vi "niRFUtil MT LTE Composite Equalization.vi"(6 "Threshold":sgl, 8 "error in (no error)":errorcluster, 9 "OFDM symbol to skip":i32, 10 "Ideal signal":csg[][](array[numeric]), 11 "Received signal":csg[][](array[numeric])) -> (0 "error out":errorcluster, 2 "Equalizer coefficients":csg[](array[numeric]), 3 "Equalized signal":csg[][](array[numeric]))   [LabVIEW 2015, in "niRFUtil.lvlib"]
uses:
  niRFUtil.lvlib
  Utilities/niRFAMT.dll
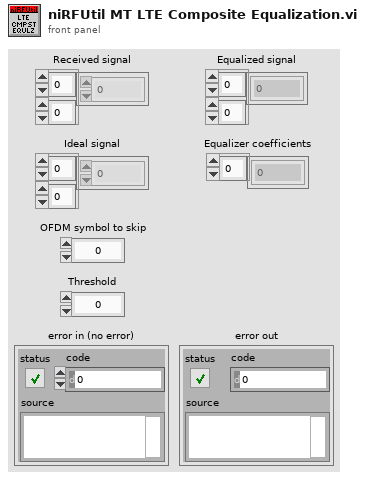
[diagram p1: front panel]
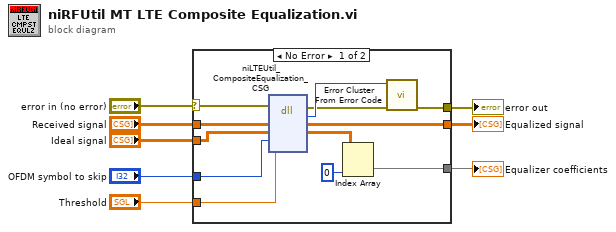
[diagram p0: block diagram]
diagram:
  n1 = case shown="No Error" "error in (no error)" {
    selector: "error in (no error)" -> [w9 w21]
    tunnel: "Received signal" -> [w20 _]
    tunnel: "Ideal signal" -> [w19 _]
    tunnel: "OFDM symbol to skip" -> [w18 _]
    tunnel: "Threshold" -> [w17 _]
    tunnel: [w16 _] -> w4
    tunnel: [w13 _] -> w3
    tunnel: [w10 w21] -> w2
    frame No Error {
      n2 = dll-call lib="C:/Perforce/semoore-sales/Customers/NATI-3813/Noise Floor/LV Filters/ParallelComplexFilterRFUtil/niRFUtil/MT/Utilities/niRFAMT.*" fn="niLTEUtil_CompositeEqualization_CSG"(error in=w9, "Received signal"=w20, "Ideal signal"=w19, "OFDM symbol to skip"=w18, "Threshold"=w17) -> (error out=w11:errorcluster, "return type"=w12:i32, "Received signal"=w16:csg[][], "Ideal signal"=w14:csg[][])  [unwired: 4 in, 1 out]
      n3 = Index Array(array=w14, index (col)=0 ("disabled index (col)")) -> (element=w13:csg[])  [unwired: 1 in]
      n4 = call <vilib>:"Error Cluster From Error Code.vi"("error in (no error)"=w11, "error code (0)"=w12) -> ("error out"=w10:errorcluster)  [unwired: 7 in]
    }
    frame Error {
    }
  }
  "Equalized signal" <- w4
  "Equalizer coefficients" <- w3
  "error out" <- w2
